vi "LCP_Arduino.vi"() -> ()   [LabVIEW 2019]
uses:
  <vilib>/Instr/_visa.llb/VISA Flush IO Buffer Mask.ctl
  <vilib>/Instr/_visa.llb/VISA Configure Serial Port (Instr).vi
panel:
  out "Offset":dbl
  in  "Scale":dbl=2049.0
  out "Index":i32
  out "Status LED":bool
  in  "Command":u16(ring) items=["MEASURE WEIGHT", "TARE", "SET SCALE", "CALIBRATION", "SHUTDOWN"]
  out "SetScale Log":string
  out "Gauge":dbl(knob) scale=0.0..1000.0
  out "Tar. Log":string
  in  "Baud Rate":u32=115200
  out "Status":string
  out "Calib. Log":string
  in  "Send Command":bool
  in  "Stop Communication":bool
  in  "Arduino port":refnum<visa-resource-name>
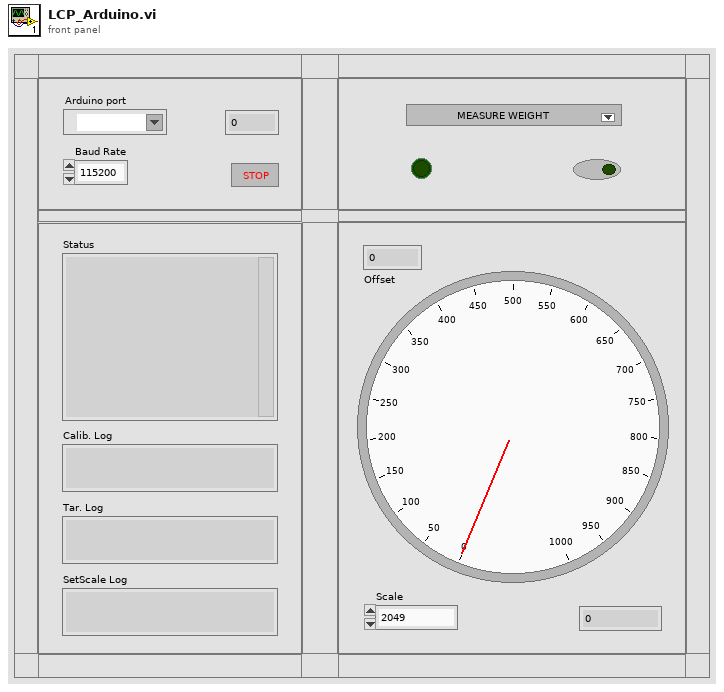
[diagram p1: front panel]
types:
  T1 = typedef "VISA Flush IO Buffer Mask.ctl" = u16
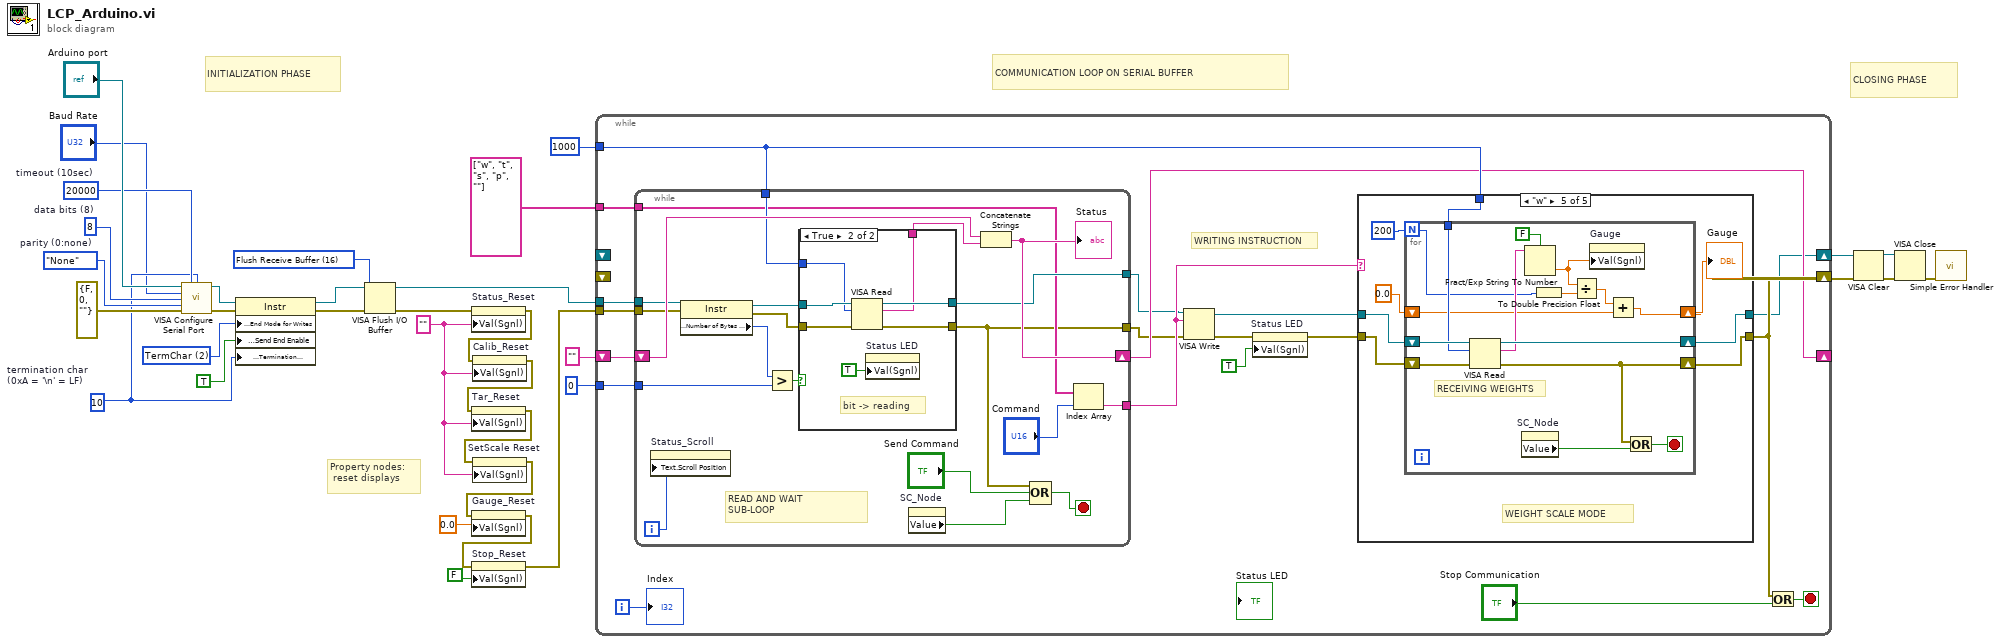
[diagram p0: block diagram]
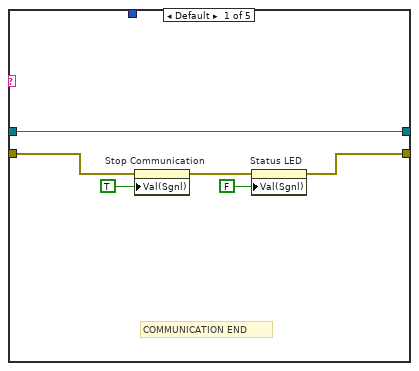
[diagram p2: hidden frame]
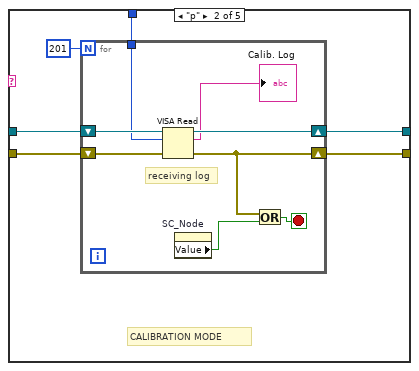
[diagram p3: hidden frame]
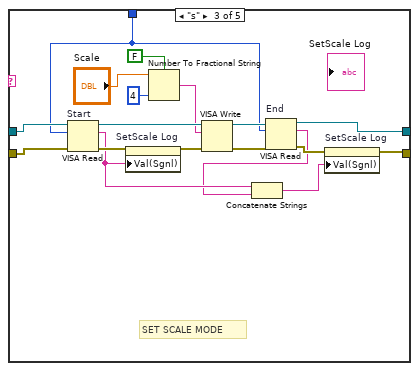
[diagram p4: hidden frame]
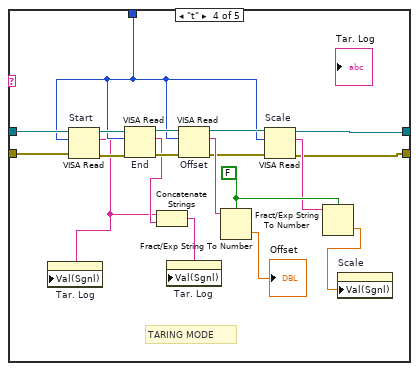
[diagram p5: hidden frame]
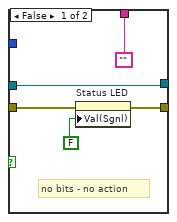
[diagram p6: hidden frame]
diagram:
  w6 = T1 16 items=["Flush Receive Buffer"=16, "Write Transmit Buffer to Device"=32, "Flush Receive Buffer (No I/O)"=64, "Flush Transmit Buffer"=128] ("Mask")
  w10 = "" ("Value (Signaling)")
  w24 = u16 2 items=["None", "Last Bit", "TermChar", "Break"] ("Serial Settings:End Mode for Writes")
  w22 = u8 10  # termination char (0xA = '\n' = LF)
  w30 = u32 20000  # timeout (10sec)
  w32 = enum16{"None", "Odd", "Even", "Mark", "Space"}."None"  # parity (0:none)
  w33 = u16 8  # data bits (8)
  # "CLOSING PHASE"
  # "COMMUNICATION LOOP ON SERIAL BUFFER"
  # "INITIALIZATION PHASE"
  # "Property nodes:\n reset displays"
  n1 = call-poly "VISA Configure Serial Port"("VISA resource name"="Arduino port", "timeout (10sec)"=w30, "termination char\n(0xA = '\\n' = LF)"=w22, "baud rate (9600)"="Baud Rate", "data bits (8)"=w33, "parity (0:none)"=w32, "error in (no error)"=errorcluster {"status"=FALSE, "code"=0, "source"=""}) -> ("VISA resource name out"=w25:refnum<visa-resource-name>, "error out"=w23:errorcluster)  [unwired: 7 in]
  n2 = property class="Instr"(reference=w25, error in=w23, "Serial Settings:End Mode for Writes"=w24, "Message Based Settings:Send End Enable"=TRUE, "Message Based Settings:Termination Character"=w22) -> (reference out=w7:refnum<visa-resource-name>, error out=w15:errorcluster)
  n3 = VISA Flush I/O Buffer(VISA resource name=w7, mask (16)=w6, error in (no error)=w15) -> (VISA resource name out=w2:refnum<visa-resource-name>, error out=w8:errorcluster)
  n4 = property on="Status_Reset" class="Str"(error in=w8, "Val(Sgnl)"=w10) -> (error out=w13:errorcluster)  [unwired: 1 in, 1 out]
  n5 = property on="Calib_Reset" class="Str"(error in=w13, "Val(Sgnl)"=w10) -> (error out=w12:errorcluster)  [unwired: 1 in, 1 out]
  n6 = property on="Tar_Reset" class="Str"(error in=w12, "Val(Sgnl)"=w10) -> (error out=w11:errorcluster)  [unwired: 1 in, 1 out]
  n7 = property on="SetScale Reset" class="Str"(error in=w11, "Val(Sgnl)"=w10) -> (error out=w1:errorcluster)  [unwired: 1 in, 1 out]
  n8 = property on="Gauge_Reset" class="Knob (strict)"(error in=w1, "Val(Sgnl)"=0.0 ("Value (Signaling)")) -> (error out=w4:errorcluster)  [unwired: 1 in, 1 out]
  n9 = property on="Stop_Reset" class="Bool (strict)"(error in=w4, "Val(Sgnl)"=FALSE ("Value (Signaling)")) -> (error out=w5:errorcluster)  [unwired: 1 in, 1 out]
  n10 = while {
    tunnel: u32 1000 ("byte count") -> [w52]
    shift-right: [w43] -> w21
    shift-left: _ -> [_]
    shift-right: [w41] -> w19
    shift-left: _ -> [_]
    tunnel: w5 -> [w45]
    tunnel: w2 -> [w51]
    shift-right: [w48] -> _
    shift-left: "" -> [w50]
    tunnel: u32 0 ("y") -> [w49]
    tunnel: string[] ["w", "t", "s", "p", ""] -> [w42]
    i -> [w39]
    stop <- w47 stop-if-true
    # "WRITING INSTRUCTION"
    n11 = while {
      shift-right: [w148] -> w48
      shift-left: w50 -> [w147]
      tunnel: w52 -> [w146]
      tunnel: [w145] -> w37
      tunnel: [w137] -> w38
      tunnel: w45 -> [w142]
      tunnel: w51 -> [w144]
      tunnel: w49 -> [w143]
      tunnel: [w139] -> w46
      tunnel: w42 -> [w140]
      i -> [w134]
      stop <- w135 stop-if-true
      # "READ AND WAIT \nSUB-LOOP"
      n12 = property on="Status_Scroll" class="Str"("Text.Scroll Position"=w134) -> ()  [unwired: 2 in, 2 out]
      n13 = property class="Instr"(reference=w144, error in=w142) -> (reference out=w151:refnum<visa-resource-name>, error out=w152:errorcluster, "Serial Settings:Number of Bytes at Serial Port"=w153:u32)
      n14 = Greater?(x=w153, y=w143) -> (0:w150:bool)
      n15 = case shown="True" w150 {
        tunnel: w152 -> [w155 w165]
        tunnel: w151 -> [w154 w164]
        tunnel: [w156 w163] -> w137
        tunnel: [w154 w162] -> w145
        tunnel: ["" w161] -> w149
        tunnel: w146 -> [_ w160]
        frame False {
          # "no bits - no action"
          n16 = property on="Status LED" class="Bool (strict)"(error in=w155, "Val(Sgnl)"=FALSE ("Value (Signaling)")) -> (error out=w156:errorcluster)  [unwired: 1 in, 1 out]
        }
        frame True {
          # "bit -> reading"
          n17 = VISA Read(VISA resource name=w164, byte count=w160, error in (no error)=w165) -> (VISA resource name out=w162:refnum<visa-resource-name>, read buffer=w161:string, error out=w163:errorcluster)  [unwired: 1 out]
          n18 = property on="Status LED" class="Bool (strict)"("Val(Sgnl)"=TRUE ("Value (Signaling)")) -> ()  [unwired: 2 in, 2 out]
        }
      }
      n19 = property on="SC_Node" class="Bool (strict)"() -> ("Value"=w136:bool)  [unwired: 2 in, 2 out]
      n20 = Concatenate Strings(w147, w149) -> (w148:string)
      "Status" <- w148
      n21 = Compound Arithmetic op=OR(w137, "Send Command", w136) -> (w135:bool)
      n22 = Index Array(array=w140, index="Command") -> (element=w139:string)
    }
    n23 = VISA Write(VISA resource name=w37, write buffer=w46, error in (no error)=w38) -> (VISA resource name out=w53:refnum<visa-resource-name>, error out=w36:errorcluster)  [unwired: 1 out]
    n24 = property on="Status LED" class="Bool (strict)"(error in=w36, "Val(Sgnl)"=TRUE ("Value (Signaling)")) -> (error out=w35:errorcluster)  [unwired: 1 in, 1 out]
    n25 = case shown="\"w\"" w46 {
      tunnel: w53 -> [w59 w65 w91 w109 w116]
      tunnel: w35 -> [w57 w64 w90 w110 w115]
      tunnel: w52 -> [_ w63 w87 w95 w112]
      tunnel: [w59 w62 w86 w101 w114] -> w41
      tunnel: [w55 w61 w81 w102 w113] -> w43
      frame Default {
        # "COMMUNICATION END"
        n26 = property on="Stop Communication" class="Bool (strict)"(error in=w57, "Val(Sgnl)"=TRUE ("Value (Signaling)")) -> (error out=w56:errorcluster)  [unwired: 1 in, 1 out]
        n27 = property on="Status LED" class="Bool (strict)"(error in=w56, "Val(Sgnl)"=FALSE ("Value (Signaling)")) -> (error out=w55:errorcluster)  [unwired: 1 in, 1 out]
      }
      frame "p" {
        # "CALIBRATION MODE"
        n28 = for {
          N: 201 -> [_]
          tunnel: w63 -> [w71]
          shift-right: [w70] -> w62
          shift-left: w65 -> [w73]
          shift-right: [w67] -> w61
          shift-left: w64 -> [w72]
          stop <- w68 stop-if-true
          # "receiving log"
          n29 = VISA Read(VISA resource name=w73, byte count=w71, error in (no error)=w72) -> (VISA resource name out=w70:refnum<visa-resource-name>, read buffer=→"Calib. Log":string, error out=w67:errorcluster)  [unwired: 1 out]
          n30 = property on="SC_Node" class="Bool (strict)"() -> ("Value"=w66:bool)  [unwired: 2 in, 2 out]
          n31 = Or(x=w67, y=w66) -> (x .or. y?=w68:bool)
        }
      }
      frame "s" {
        # "SET SCALE MODE"
        n32 = VISA Read "Start"(VISA resource name=w91, byte count=w87, error in (no error)=w90) -> (VISA resource name out=w89:refnum<visa-resource-name>, read buffer=w80:string, error out=w84:errorcluster)  [unwired: 1 out]
        n33 = property on="SetScale Log" class="Str"(error in=w84, "Val(Sgnl)"=w80) -> (error out=w83:errorcluster)  [unwired: 1 in, 1 out]
        n34 = Number To Fractional String(use system decimal point (T)=FALSE, number="Scale", precision (6)=i16 4) -> (F-format string=w77:string)  [unwired: 1 in]
        n35 = VISA Write(VISA resource name=w89, write buffer=w77, error in (no error)=w83) -> (VISA resource name out=w88:refnum<visa-resource-name>, error out=w85:errorcluster)  [unwired: 1 out]
        n36 = VISA Read "End"(VISA resource name=w88, byte count=w87, error in (no error)=w85) -> (VISA resource name out=w86:refnum<visa-resource-name>, read buffer=w79:string, error out=w82:errorcluster)  [unwired: 1 out]
        n37 = Concatenate Strings(w80, w79) -> (w78:string)
        n38 = property on="SetScale Log" class="Str"(error in=w82, "Val(Sgnl)"=w78) -> (error out=w81:errorcluster)  [unwired: 1 in, 1 out]
      }
      frame "t" {
        w108 = FALSE ("use system decimal point (T)")
        # "TARING MODE"
        n39 = VISA Read "Start"(VISA resource name=w109, byte count=w95, error in (no error)=w110) -> (VISA resource name out=w97:refnum<visa-resource-name>, read buffer=w93:string, error out=w99:errorcluster)  [unwired: 1 out]
        n40 = property on="Tar. Log" class="Str"("Val(Sgnl)"=w93) -> ()  [unwired: 2 in, 2 out]
        n41 = VISA Read "End"(VISA resource name=w97, byte count=w95, error in (no error)=w99) -> (VISA resource name out=w96:refnum<visa-resource-name>, read buffer=w94:string, error out=w98:errorcluster)  [unwired: 1 out]
        n42 = Concatenate Strings(w93, w94) -> (w92:string)
        n43 = property on="Tar. Log" class="Str"("Val(Sgnl)"=w92) -> ()  [unwired: 2 in, 2 out]
        n44 = VISA Read "Offset"(VISA resource name=w96, byte count=w95, error in (no error)=w98) -> (VISA resource name out=w104:refnum<visa-resource-name>, read buffer=w106:string, error out=w105:errorcluster)  [unwired: 1 out]
        n45 = Fract/Exp String To Number(use system decimal point (T)=w108, string=w106) -> (number=→"Offset":dbl)  [unwired: 2 in, 1 out]
        n46 = VISA Read "Scale"(VISA resource name=w104, byte count=w95, error in (no error)=w105) -> (VISA resource name out=w101:refnum<visa-resource-name>, read buffer=w107:string, error out=w102:errorcluster)  [unwired: 1 out]
        n47 = Fract/Exp String To Number(use system decimal point (T)=w108, string=w107) -> (number=w100:dbl)  [unwired: 2 in, 1 out]
        n48 = property on="Scale" class="DigNum (strict)"("Val(Sgnl)"=w100) -> ()  [unwired: 2 in, 2 out]
      }
      frame "w" {
        # "WEIGHT SCALE MODE"
        n49 = for {
          N: 200 -> [w124]
          tunnel: w112 -> [w131]
          shift-right: [w130] -> w114
          shift-left: w116 -> [w133]
          shift-right: [w128] -> w113
          shift-left: w115 -> [w132]
          shift-right: [w119] -> w111
          shift-left: 0.0 -> [w125]
          stop <- w127 stop-if-true
          # "RECEIVING WEIGHTS"
          n50 = VISA Read(VISA resource name=w133, byte count=w131, error in (no error)=w132) -> (VISA resource name out=w130:refnum<visa-resource-name>, read buffer=w129:string, error out=w128:errorcluster)  [unwired: 1 out]
          n51 = property on="SC_Node" class="Bool (strict)"() -> ("Value"=w122:bool)  [unwired: 2 in, 2 out]
          n52 = Fract/Exp String To Number(use system decimal point (T)=FALSE, string=w129) -> (number=w120:dbl)  [unwired: 2 in, 1 out]
          n53 = To Double Precision Float(number=w124) -> (double precision float=w123:dbl)
          n54 = Divide(x=w120, y=w123) -> (x/y=w126:dbl)
          n55 = property on="Gauge" class="Knob (strict)"("Val(Sgnl)"=w120) -> ()  [unwired: 2 in, 2 out]
          n56 = Add(x=w126, y=w125) -> (x+y=w119:dbl)
          n57 = Or(x=w128, y=w122) -> (x .or. y?=w127:bool)
        }
        "Gauge" <- w111
      }
    }
    n58 = Or(x=w43, y="Stop Communication") -> (x .or. y?=w47:bool)
    "Index" <- w39
  }
  n59 = VISA Clear(VISA resource name=w19, error in (no error)=w21) -> (VISA resource name out=w28:refnum<visa-resource-name>, error out=w29:errorcluster)
  n60 = VISA Close(VISA resource name=w28, error in (no error)=w29) -> (error out=w27:errorcluster)
  n61 = call <vilib>:"Simple Error Handler.vi"("error in (no error)"=w27) -> ()  [unwired: 4 in, 5 out]
